vi "PCSLauncher.ProcEvents.vi"(0 "i ref in":refnum<vi>, 5 "error in (no error)":errorcluster) -> (14 "i ref out":refnum<vi>, 19 "error out":errorcluster)   [LabVIEW 2014, in "PCSLauncher.lvlib"]
doc: "This method is used to define the events the object will listen to. Add your own events here."
uses:
  PCSLauncher.lvlib
  CSCore/BaseProcess/BaseProcess.lvlib
  PH_Common/PH_Common.lvlib
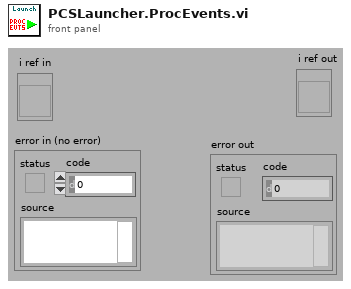
[diagram p1: front panel]
types:
  T1 = typedef "PH_Common.lvlib/PH_DIM.Event Declarer.ctl" = cluster{"Service Name":string, "Selector":string}
  T2 = typedef "BaseProcess.lvlib/BaseProcess.event definition.ctl" = cluster{"CAEEvtDef":T3, "Data Descriptor":T4}
  T3 = typedef "CAEObj.lvlib/CAEObj.event definition.ctl" = cluster{"URL":string, "enable":bool, "ignoreResID":bool}
  T4 = typedef "BaseProcess.lvlib/BaseProcess.descriptor string definition.ctl" = string
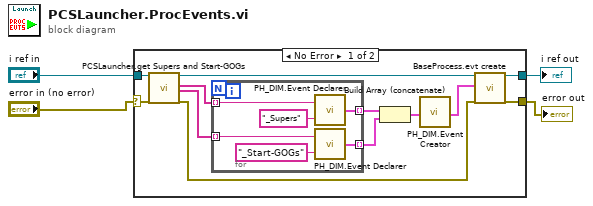
[diagram p0: block diagram]
diagram:
  n1 = case shown="No Error" "error in (no error)" {
    selector: "error in (no error)" -> [w14 w23]
    tunnel: "i ref in" -> [w13 w24]
    tunnel: [w16 w23] -> w3
    tunnel: [w15 w24] -> w2
    frame No Error {
      n2 = call "PCSLauncher.get Supers and Start-GOGs.vi"("i ref in"=w13, "error in (no error)"=w14) -> ("i ref out"=w12:refnum<vi>, "Super Instances"=w9:string[], "Start-GOG Instances"=w8:string[], "error out"=w5:errorcluster)  [unwired: 13 in, 1 out]
      n3 = for {
        tunnel: [w20] -> w7 mode=indexing
        tunnel: [w19] -> w6 mode=indexing
        tunnel: w9 -> [w18] mode=indexing
        tunnel: w8 -> [w17] mode=indexing
        n4 = call "PH_DIM.Event Declarer.vi"("Selector"="_Supers", "Service Name"=w18) -> ("declared DIM Event"=w20:T1)
        n5 = call "PH_DIM.Event Declarer.vi"("Selector"="_Start-GOGs", "Service Name"=w17) -> ("declared DIM Event"=w19:T1)
      }
      n6 = Build Array (concatenate)(w7, w6) -> (w10:T1[])
      n7 = call "PH_DIM.Event Creator.vi"("condition Services"=w10) -> ("DIM Service Events"=w11:T2[])  [unwired: 18 in]
      n8 = call "BaseProcess.evt create.vi"("i ref in"=w12, "newEvents"=w11, "error in (no error)"=w5) -> ("i ref out"=w15:refnum<vi>, "error out"=w16:errorcluster)  [unwired: 13 in, 2 out]
    }
    frame Error {
    }
  }
  "i ref out" <- w2
  "error out" <- w3
